vi "getAttachmentPoint.vi"(0 "reference":refnum<class "StateTransitionEdge.lvclass">, 1 "graphics":refnum<class "Graphics.lvclass">, 2 "p1":T1 {"y" format="%.2f"; "x" format="%.2f"}, 3 "p2":T1 {"y" format="%.2f"; "x" format="%.2f"}, 4 "text":string, 5 "error in (no error)":errorcluster, 7 "center":bool) -> (14 "reference out":refnum<class "StateTransitionEdge.lvclass">, 15 "attachPoint":T1 {"y" format="%.2f"; "x" format="%.2f"}, 19 "error out":errorcluster)   [LabVIEW 2012, in "StateTransitionEdge.lvclass"]
doc: "\"private static Point2D getAttachmentPoint(Graphics2D g2,"
uses:
  <resource>/Framework/Providers/Open_GDS/UML/StateTransitionEdge_class/StateTransitionEdge.lvclass
  <resource>/Framework/Providers/Open_GDS/UML/General/Point/Point Point2D.ctl
  <resource>/Framework/Providers/Open_GDS/UML/Graphics_class/Graphics.lvclass
  <resource>/Framework/Providers/Open_GDS/UML/General/Rectangle/Rectangle Rectangle2D.ctl
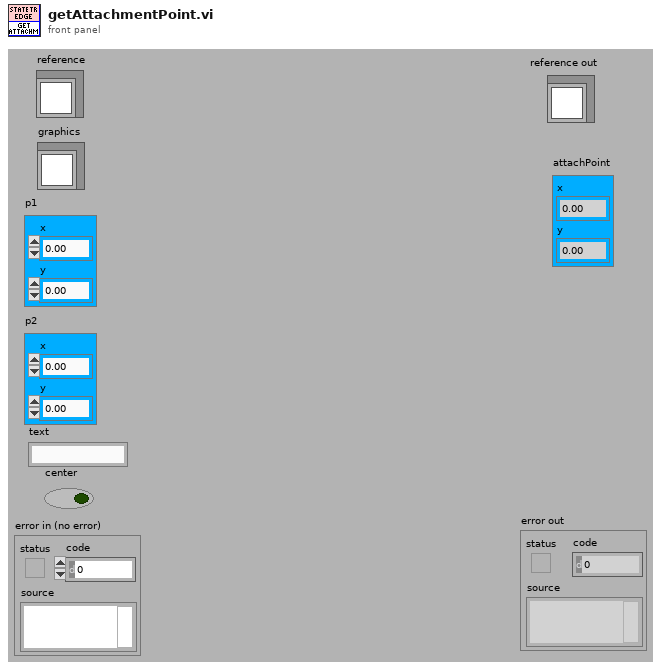
[diagram p1: front panel]
types:
  T1 = typedef "Point Point2D.ctl" = cluster{"x":dbl, "y":dbl}
  T2 = typedef "Rectangle Rectangle2D.ctl" = cluster{"x":dbl, "y":dbl, "width":dbl, "height":dbl}
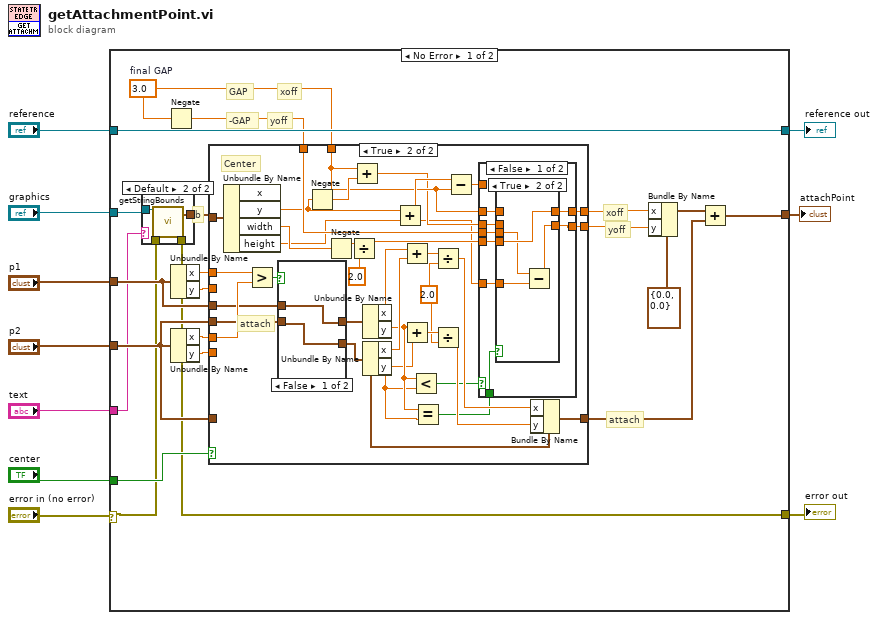
[diagram p0: block diagram]
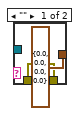
[diagram p2: hidden frame]
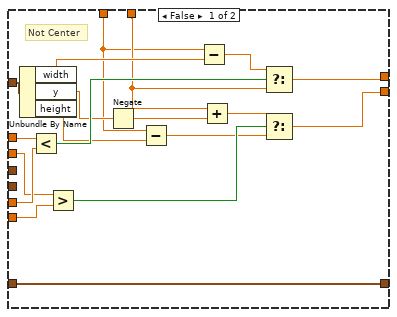
[diagram p3: hidden frame]
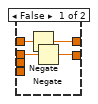
[diagram p4: hidden frame]
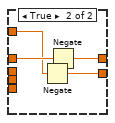
[diagram p5: hidden frame]
diagram:
  n1 = case shown="No Error" "error in (no error)" {
    selector: "error in (no error)" -> [w13 w115]
    tunnel: "reference" -> [w29 w116]
    tunnel: [w12 w115] -> w9
    tunnel: [w29 w116] -> w8
    tunnel: "graphics" -> [w15 _]
    tunnel: "text" -> [w14 _]
    tunnel: [w20 _] -> w4
    tunnel: "center" -> [w30 _]
    tunnel: "p1" -> [w26 _]
    tunnel: "p2" -> [w23 _]
    frame No Error {
      w25 = 3.0  # final GAP
      # "yoff"
      # "xoff"
      # "attach"
      # "yoff"
      # "xoff"
      # "GAP"
      # "-GAP"
      n2 = case shown="Default" w14 {
        tunnel: w15 -> [_ w37]
        tunnel: w13 -> [w32 w36]
        tunnel: [T2 {"x"=0.0, "y"=0.0, "width"=0.0, "height"=0.0} ("bounds") w35] -> w11
        tunnel: [w32 w34] -> w12
        frame "" {
        }
        frame Default {
          # "b"
          n3 = call-dynamic "getStringBounds.vi"("reference"=w37, "error in (no error)"=w36) -> ("bounds"=w35:T2, "error out"=w34:errorcluster)  [unwired: 3 in, 13 out]
        }
      }
      n4 = Negate(x=w25) -> (-x=w24:dbl)
      n5 = Unbundle By Name(w26) -> ("x"=w28:dbl, "y"=w17:dbl)
      n6 = Unbundle By Name(w23) -> ("x"=w27:dbl, "y"=w16:dbl)
      n7 = case shown="True" w30 {
        tunnel: w28 -> [w56 w90]
        tunnel: w27 -> [w55 w89]
        tunnel: w26 -> [_ w87]
        tunnel: w23 -> [_ w86]
        tunnel: w24 -> [w40 w66]
        tunnel: w25 -> [w46 w59]
        tunnel: w23 -> [w54 _]
        tunnel: [w54 w78] -> w21
        tunnel: [w44 w73] -> w19
        tunnel: [w52 w67] -> w18
        tunnel: w11 -> [w51 w75]
        tunnel: w17 -> [w43 _]
        tunnel: w16 -> [w42 _]
        frame False {
          # "Not Center"
          n8 = Unbundle By Name(w51) -> ("width"=w50:dbl, "y"=w48:dbl, "height"=w38:dbl)
          n9 = Less?(x=w56, y=w55) -> (x < y?=w53:bool)
          n10 = Greater?(x=w43, y=w42) -> (0:w41:bool)
          n11 = Negate(x=w48) -> (-x=w47:dbl)
          n12 = Subtract(x=w40, y=w38) -> (x-y=w39:dbl)
          n13 = Subtract(x=w40, y=w50) -> (x-y=w49:dbl)
          n14 = Add(x=w46, y=w47) -> (x+y=w45:dbl)
          n15 = Select(t=w49, s=w53, f=w46) -> (s? t:f=w52:dbl)
          n16 = Select(t=w45, s=w41, f=w39) -> (s? t:f=w44:dbl)
        }
        frame True {
          w80 = 2.0 ("y")
          # "attach"
          # "Center"
          n17 = Unbundle By Name(w75) -> ("y"=w61:dbl, "width"=w64:dbl, "height"=w57:dbl)  [unwired: 1 out]
          n18 = Greater?(x=w90, y=w89) -> (0:w88:bool)
          n19 = case shown="False" w88 {
            tunnel: w87 -> [w112 w114]
            tunnel: [w111 w114] -> w79
            tunnel: [w112 w113] -> w85
            tunnel: w86 -> [w111 w113]
            frame False {
            }
            frame True {
            }
          }
          n20 = Negate(x=w61) -> (-x=w60:dbl)
          n21 = Negate(x=w64) -> (-x=w63:dbl)
          n22 = Divide(x=w63, y=2.0) -> (x/y=w62:dbl)
          n23 = Add(x=w59, y=w60) -> (x+y=w58:dbl)
          n24 = Unbundle By Name(w85) -> ("x"=w84:dbl, "y"=w70:dbl)
          n25 = Unbundle By Name(w79) -> ("x"=w83:dbl, "y"=w69:dbl)
          n26 = Add(x=w61, y=w57) -> (x+y=w74:dbl)
          n27 = Add(x=w84, y=w83) -> (x+y=w82:dbl)
          n28 = Add(x=w70, y=w69) -> (x+y=w81:dbl)
          n29 = Less?(x=w70, y=w69) -> (x < y?=w71:bool)
          n30 = Equal?(x=w70, y=w69) -> (x = y?=w68:bool)
          n31 = Divide(x=w82, y=w80) -> (x/y=w77:dbl)
          n32 = Divide(x=w81, y=w80) -> (x/y=w76:dbl)
          n33 = Subtract(x=w74, y=w59) -> (x-y=w72:dbl)
          n34 = case shown="False" w71 {
            tunnel: [w97 w108] -> w73
            tunnel: w72 -> [_ w109]
            tunnel: w68 -> [w98 _]
            tunnel: w59 -> [w93 w110]
            tunnel: [w95 w107] -> w67
            tunnel: w66 -> [w96 _]
            tunnel: w62 -> [w94 _]
            tunnel: w58 -> [w92 _]
            tunnel: w57 -> [w91 _]
            frame False {
              n35 = case shown="True" w98 {
                tunnel: [w100 w103] -> w97
                tunnel: w96 -> [_ w104]
                tunnel: [w99 w106] -> w95
                tunnel: w94 -> [_ w106]
                tunnel: w93 -> [w102 _]
                tunnel: w92 -> [w101 _]
                tunnel: w91 -> [_ w105]
                frame False {
                  n36 = Negate(x=w102) -> (-x=w99:dbl)
                  n37 = Negate(x=w101) -> (-x=w100:dbl)
                }
                frame True {
                  n38 = Subtract(x=w104, y=w105) -> (x-y=w103:dbl)
                }
              }
            }
            frame True {
              n39 = Negate(x=w109) -> (-x=w108:dbl)
              n40 = Negate(x=w110) -> (-x=w107:dbl)
            }
          }
          n41 = Bundle By Name(cluster=w79, "x"=w77, "y"=w76) -> (w78:T1)
        }
      }
      n42 = Bundle By Name(cluster=T1 {"x"=0.0, "y"=0.0} ("attachPoint"), "x"=w18, "y"=w19) -> (w22:T1)
      n43 = Add(x=w22, y=w21) -> (x+y=w20:T1)
    }
    frame Error {
    }
  }
  "reference out" <- w8
  "error out" <- w9
  "attachPoint" <- w4
